vi "rqcAlice Attenuator Test (Host).vi"() -> ()   [LabVIEW 2018]
uses:
  Alice Host Library/Low Level/SPI/SPI.SubVIs/SPI.SubSystem.ctl
  <vilib>/FPGAPlugInAG/PCIe-7820R/niLvFpga_Open_PCIe-7820R.vi
  <vilib>/rvi/interface/common/dynamic/niFpgaDynamicAddResources.vi
  <vilib>/FPGAPlugInAG/Dynamic/niLvFpga_Close_Dynamic.vi
  <vilib>/rvi/interface/nirviOpenFPGA/nirviOpenFPGA.xnode
  FPGA Bitfiles/rqcAlice FPGA (7820R) v 2.3.0.lvbitx
  <vilib>/rvi/interface/nirviCloseFPGA/nirviCloseFPGA.xnode
  Automated Measurements/KeySight 8164B LAN InstrLib.lvlib
panel:
  in  "write to file":bool
  in  "Raw value":bool
  in  "start value":u16
  in  "Base Power value":dbl=7.782
  out "XY Graph":cluster{dbl[], dbl[]}[](graph)
  out "Current Attenuation":dbl
  out "Current Value":dbl
  in  "DAC Max Value":u16=225
  out "error out":errorcluster
  in  "stop":bool
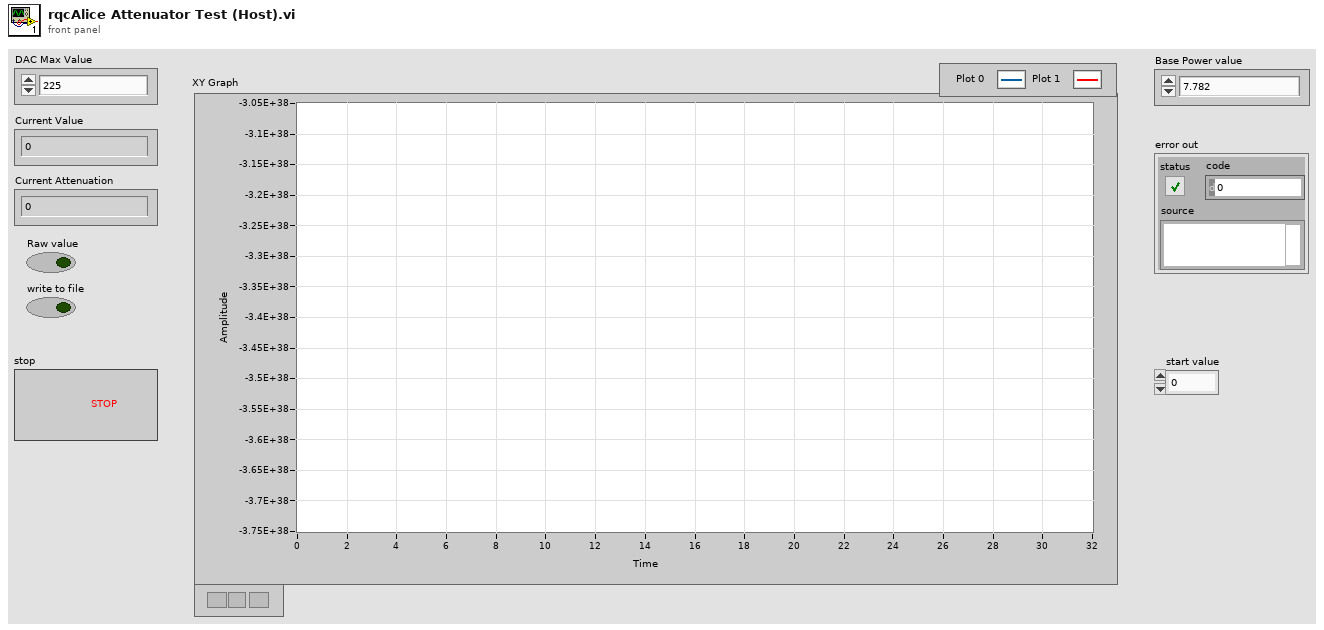
[diagram p1: front panel]
types:
  T1 = typedef "SPI.SubSystem.ctl" = enum8{"N/A", "DelayLine.MSB", "DelayLine.LSB", "Attenuation.dB", "Attenuation.DAC value"}
  T2 = enum16{"open", "replace", "create", "open or create", "replace or create", "replace or create with confirmation"}
  T3 = typedef "KeySight 8164B LAN InstrLib.lvlib/KeySight 8164B control.ctl" = cluster{"Connection ID":refnum<k5>, "Connected":bool, "Info":string, "Slots Info":string[]}
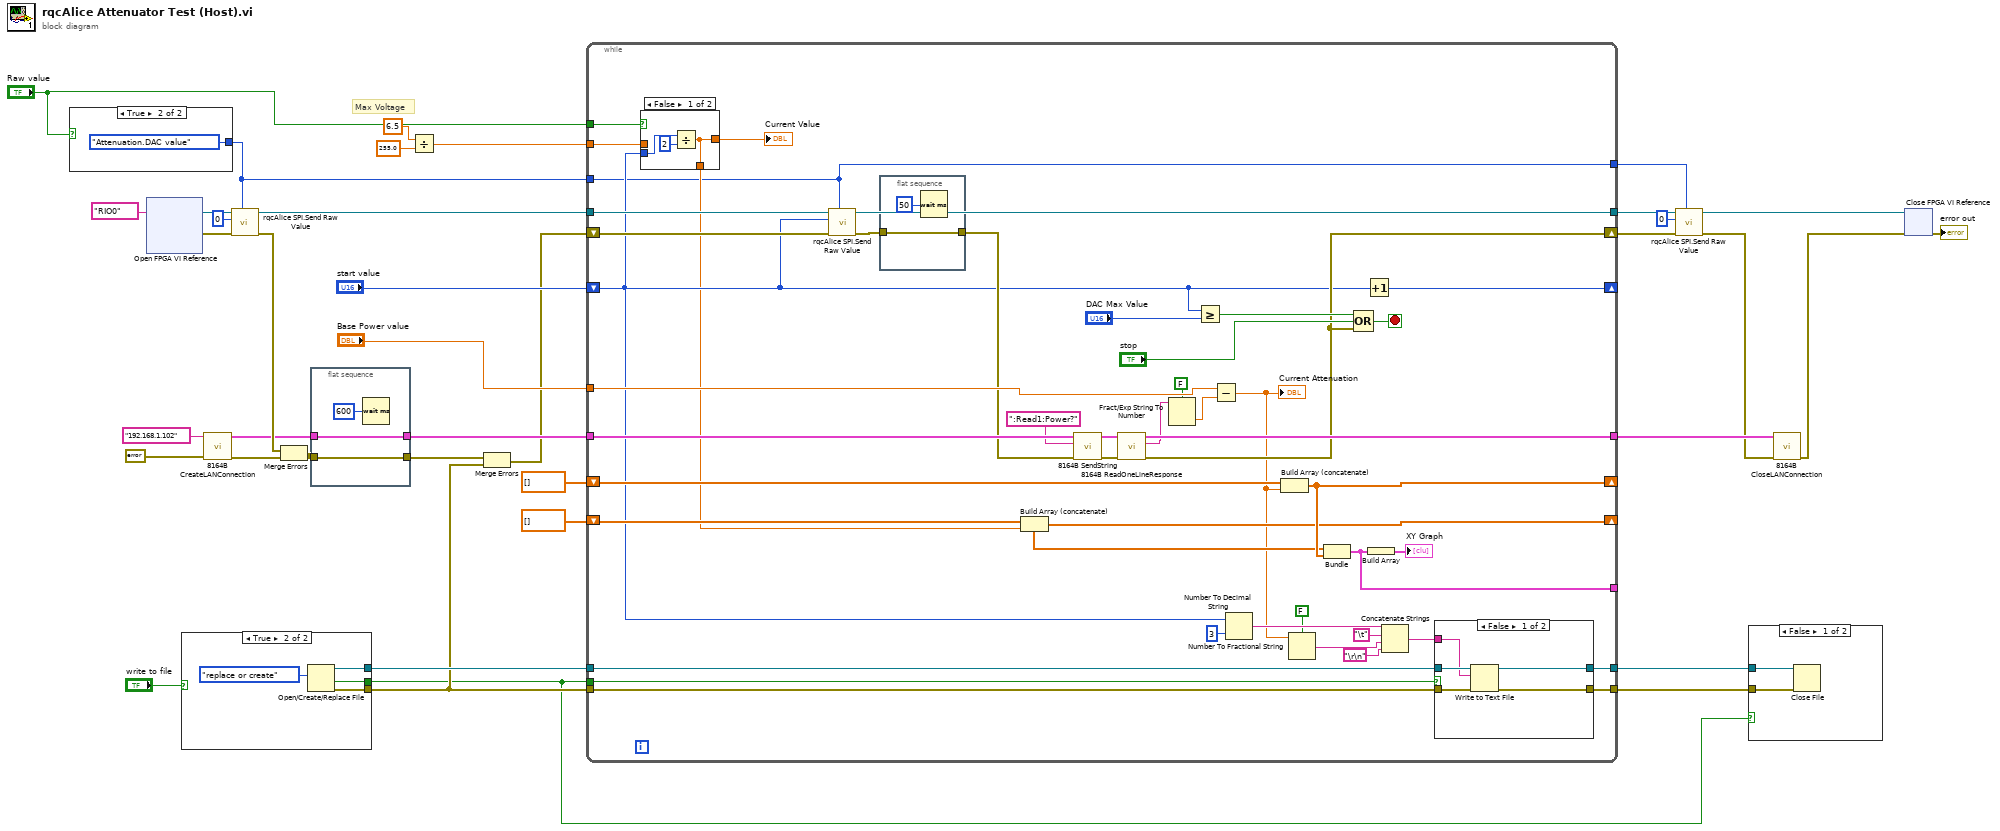
[diagram p0: block diagram]
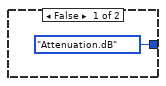
[diagram p2: hidden frame]
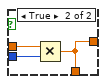
[diagram p3: hidden frame]
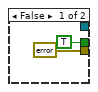
[diagram p5: hidden frame]
diagram:
  # "Max Voltage"
  n1 = case shown="True" "Raw value" {
    tunnel: [SPI.SubSystem."Attenuation.dB" ("SPI.subSystem") SPI.SubSystem."Attenuation.DAC value" ("SPI.subSystem")] -> w21
    frame False {
    }
    frame True {
    }
  }
  n2 = xnode "Open FPGA VI Reference"("resource name"=tag "RIO0") -> ("FPGA VI Reference Out"=w33:refnum<k20>, "error out"=w32:errorcluster)  [unwired: 1 in]
  n3 = case shown="True" "write to file" {
    tunnel: [_ w46] -> w14
    tunnel: [TRUE ("cancelled") w45] -> w9
    tunnel: [errorcluster {"status"=FALSE, "code"=0, "source"=""} ("error out") w44] -> w12
    frame False {
    }
    frame True {
      n4 = Open/Create/Replace File(operation (0:open)=T2."replace or create") -> (refnum out=w46:refnum<file>, cancelled=w45:bool, error out=w44:errorcluster)  [unwired: 5 in]
    }
  }
  n5 = call "8164B CreateLANConnection.vi"("error in"=errorcluster {"status"=FALSE, "code"=0, "source"=""}, "IP address"="192.168.1.102" ("address")) -> ("error out"=w15:errorcluster, "KeySight 8164B control out"=w16:T3)  [unwired: 8 in]
  n6 = call "rqcAlice SPI.Send Raw Value.vi"("SPI.subSystem"=w21, "error in"=w32, "value"=u16 0, "Alice FPGA Reference In"=w33) -> ("error out"=w18:errorcluster, "Alice FPGA Reference Out"=w30:refnum<k20>)  [unwired: 6 in]
  n7 = Merge Errors(w18, w15) -> (w19:errorcluster)
  n8 = flat-sequence {
    tunnel: [w49] -> w22
    tunnel: w16 -> [w49]
    tunnel: [w48] -> w20
    tunnel: w19 -> [w48]
    frame #0 {
      n9 = Wait (ms)(milliseconds to wait=u32 600) -> ()  [unwired: 1 out]
    }
  }
  n10 = Divide(x=6.5, y=255.0) -> (x/y=w27:dbl)
  n11 = Merge Errors(w20, w12) -> (w13:errorcluster)
  n12 = while {
    tunnel: w30 -> [w93]
    shift-right: [w83] -> w4
    shift-left: w13 -> [w92]
    tunnel: [w91] -> w8
    tunnel: "Base Power value" -> [w82]
    tunnel: w22 -> [w90]
    shift-right: [w89] -> _
    shift-left: "start value" -> [w60]
    tunnel: w27 -> [w86]
    tunnel: [w85] -> w26
    shift-right: [w79] -> _
    shift-left: dbl[] [] -> [w81]
    shift-right: [w78] -> _
    shift-left: dbl[] [] -> [w80]
    tunnel: w21 -> [w57]
    tunnel: w14 -> [w75]
    tunnel: w12 -> [w74]
    tunnel: w9 -> [w73]
    tunnel: [w65] -> w2
    tunnel: [w64] -> w1
    tunnel: "Raw value" -> [w63]
    tunnel: [w59] -> _
    tunnel: [w57] -> w6
    stop <- w94 stop-if-true
    n13 = case shown="False" w63 {
      tunnel: w86 -> [_ w100]
      tunnel: [w96 w98] -> w58
      tunnel: w60 -> [w97 w99]
      tunnel: [w96 w98] -> w62
      frame False {
        n14 = Divide(x=w97, y=u16 2) -> (x/y=w96:dbl)
      }
      frame True {
        n15 = Multiply(x=w100, y=w99) -> (x*y=w98:dbl)
      }
    }
    "Current Value" <- w62
    n16 = call "rqcAlice SPI.Send Raw Value.vi"("SPI.subSystem"=w57, "error in"=w92, "value"=w60, "Alice FPGA Reference In"=w93) -> ("error out"=w77:errorcluster, "Alice FPGA Reference Out"=w91:refnum<k20>)  [unwired: 6 in]
    n17 = flat-sequence {
      tunnel: w77 -> [w102]
      tunnel: [w102] -> w76
      frame #0 {
        n18 = Wait (ms)(milliseconds to wait=u32 50) -> ()  [unwired: 1 out]
      }
    }
    n19 = Build Array (concatenate)(w80, w58) -> (w78:dbl[])
    n20 = call "8164B SendString.vi"("error in"=w76, "CMD"=":Read1:Power?", "KeySight 8164B control in"=w90) -> ("error out"=w54:errorcluster, "KeySight 8164B control out"=w56:T3)  [unwired: 7 in]
    n21 = call "8164B ReadOneLineResponse.vi"("error in"=w54, "KeySight 8164B control in"=w56) -> ("error out"=w83:errorcluster, "OneLineResponse"=w52:string, "KeySight 8164B control out"=w85:T3)  [unwired: 7 in]
    n22 = Fract/Exp String To Number(use system decimal point (T)=FALSE, string=w52) -> (number=w51:dbl)  [unwired: 2 in, 1 out]
    n23 = Greater Or Equal?(x=w60, y="DAC Max Value") -> (x >= y?=w87:bool)
    n24 = Subtract(x=w82, y=w51) -> (x-y=w50:dbl)
    "Current Attenuation" <- w50
    n25 = Number To Decimal String(number=w60, width (-)=i16 3) -> (decimal integer string=w71:string)
    n26 = Build Array (concatenate)(w81, w50) -> (w79:dbl[])
    n27 = Number To Fractional String(use system decimal point (T)=FALSE, number=w50) -> (F-format string=w68:string)  [unwired: 2 in]
    n28 = Bundle(w78, w79) -> (w59:cluster{dbl[], dbl[]})  [unwired: 1 in]
    n29 = Compound Arithmetic op=OR(w87, "stop", w83) -> (w94:bool)
    n30 = Increment(x=w60) -> (x+1=w89:u16)
    n31 = Build Array(w59) -> (→"XY Graph":cluster{dbl[], dbl[]}[])
    n32 = Concatenate Strings(w71, "\t", w68, "\r\n") -> (w66:string)
    n33 = case shown="False" w73 {
      tunnel: w75 -> [w107 w109]
      tunnel: w74 -> [w106 w108]
      tunnel: w66 -> [w105 _]
      tunnel: [w104 w109] -> w65
      tunnel: [w103 w108] -> w64
      frame False {
        n34 = Write to Text File(file (use dialog)=w107, text=w105, error in=w106) -> (refnum out=w104:refnum<file>, error out=w103:errorcluster)  [unwired: 1 in, 1 out]
      }
      frame True {
      }
    }
  }
  n35 = call "rqcAlice SPI.Send Raw Value.vi"("SPI.subSystem"=w6, "error in"=w4, "value"=u16 0, "Alice FPGA Reference In"=w8) -> ("error out"=w3:errorcluster, "Alice FPGA Reference Out"=w7:refnum<k20>)  [unwired: 6 in]
  n36 = case shown="False" w9 {
    tunnel: w2 -> [w111 _]
    tunnel: w1 -> [w110 _]
    frame False {
      n37 = Close File(refnum=w111, error in=w110) -> ()  [unwired: 2 out]
    }
    frame True {
    }
  }
  n38 = call "8164B CloseLANConnection.vi"("error in"=w3, "KeySight 8164B control"=w26) -> ("error out"=w31:errorcluster)  [unwired: 9 in]
  n39 = xnode "Close FPGA VI Reference"("FPGA VI Reference In"=w7, "error in"=w31) -> ("error out"=→"error out":errorcluster)
